vi "Read and Calc Analog.vi"() -> ()   [LabVIEW 2013]
panel:
  out "Результат измерений":string
  in  "Знаков после запятой":i32
  out "Относительная погрешность, %":dbl
  out "Абсолютная погрешность, В":dbl
  in  "Класс точности":dbl
  out "Диапазон\nизмерений, В":dbl
  out "Показания\nвольтметра, В":dbl
  out "Шкала вольтметра":dbl(knob) scale=0.0..150.0
  in  "Выбор предела измерений":i32(knob)=8 min=0 max=8 step=1 scale=0.0..8.0
  in  "Вариант":T1(ring)
  # "Обработка показаний аналогового вольтметра"
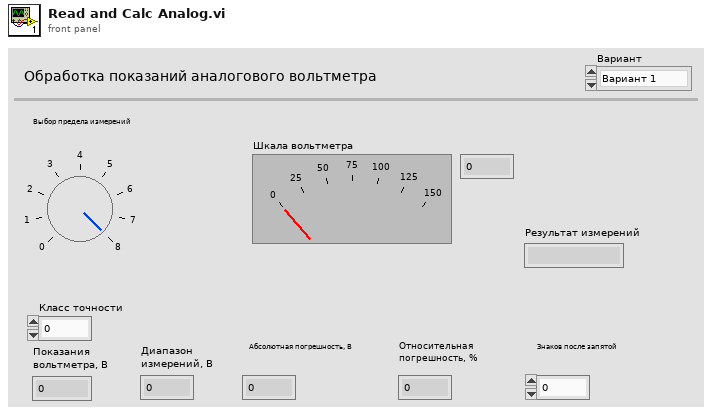
[diagram p1: front panel]
types:
  T1 = enum16{"Вариант 1", "Вариант 2", "Вариант 3", "Вариант 4", "Вариант 5", "Вариант 6", "Вариант 7", "Вариант 8", "Вариант 9", "Вариант 10", "Вариант 11", "Вариант 12"}
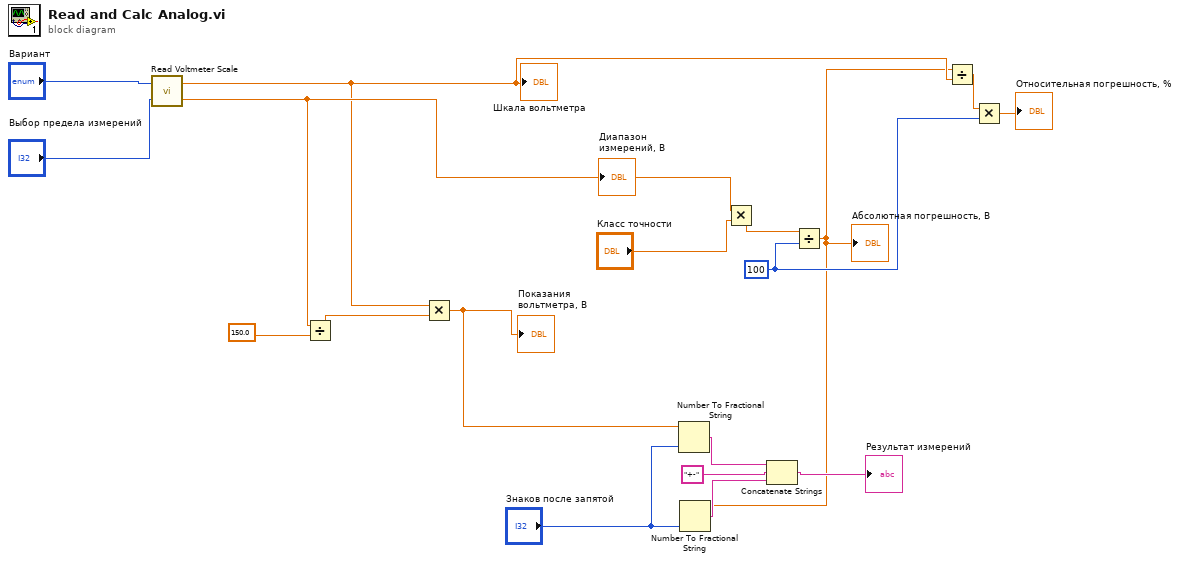
[diagram p0: block diagram]
diagram:
  w9 = 100
  n1 = call "Read Voltmeter Scale.vi"("Предел"="Выбор предела измерений", "Вариант"="Вариант") -> ("Установленный предел"=w14:dbl, "Положение указателя"=w11:dbl)
  "Шкала вольтметра" <- w11
  "Диапазон\nизмерений, В" <- w14
  n2 = Divide(x=w14, y=150.0) -> (x/y=w15:dbl)
  n3 = Multiply(x=w11, y=w15) -> (x*y=w2:dbl)
  "Показания\nвольтметра, В" <- w2
  n4 = Number To Fractional String(number=w2, precision (6)="Знаков после запятой") -> (F-format string=w5:string)  [unwired: 2 in]
  n5 = Multiply(x=w14, y="Класс точности") -> (x*y=w12:dbl)
  n6 = Divide(x=w12, y=w9) -> (x/y=w1:dbl)
  "Абсолютная погрешность, В" <- w1
  n7 = Number To Fractional String(number=w1, precision (6)="Знаков после запятой") -> (F-format string=w4:string)  [unwired: 2 in]
  n8 = Concatenate Strings(w5, "+-", w4) -> (→"Результат измерений":string)
  n9 = Divide(x=w1, y=w11) -> (x/y=w10:dbl)
  n10 = Multiply(x=w10, y=w9) -> (x*y=→"Относительная погрешность, %":dbl)
